vi "AssertControlValue [Poly].vi"   [LabVIEW 2016]
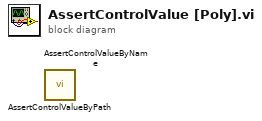
[diagram p0: block diagram]
diagram:
  n1 = call "AssertControlValueByPath.vi"() -> ()  [unwired: 13 in, 3 out]
  n2 = call "AssertControlValueByName.vi"() -> ()  [unwired: 13 in, 3 out]
